vi "Wind Farm #3.vi"(8 "error in (no error)":errorcluster) -> (0 "error out":errorcluster)   [LabVIEW 2011]
doc: "This is one of 4 potential implementations for the Wind Farm Requirements. Specifically note how the wind turbine information is displayed. Also note how the main VI communicates back and forth to the wind turbine. What does that pipeline look like? Finally note the mechanism for stopping the wind turbine.\n\nAAL 9/09"
uses:
  Controls/File Type.ctl
  Controls/TYPE FGV User Event Method.ctl
  SEQ Solution/Controls/Wind Turbine DataRef.ctl
  SEQ Solution/Controls/Wind Turbine Data.ctl
  Shared/QDMH Poly VIs/QDMH POLY Enqueue String.vi
  SEQ Solution/SEQ - Solution.lvlib
panel:
  out "Wind Turbine Data":string[][](table)
  in  "File Type":T1 caption="File Type (Read When Turbine is Added)"
  in  "Set Wind Speed":bool
  in  "Wind Speed":dbl=15.0
  in  "Wind Turbine Selection":u16(ring)
  in  "Queue Name":string
  in  "Add Wind Turbine":bool
  out "Message Display":string
  in  "Exit":bool
  # "Rotation (RPM)"
  # "Wind Speed (m/s)"
  # "Running Time (sec)"
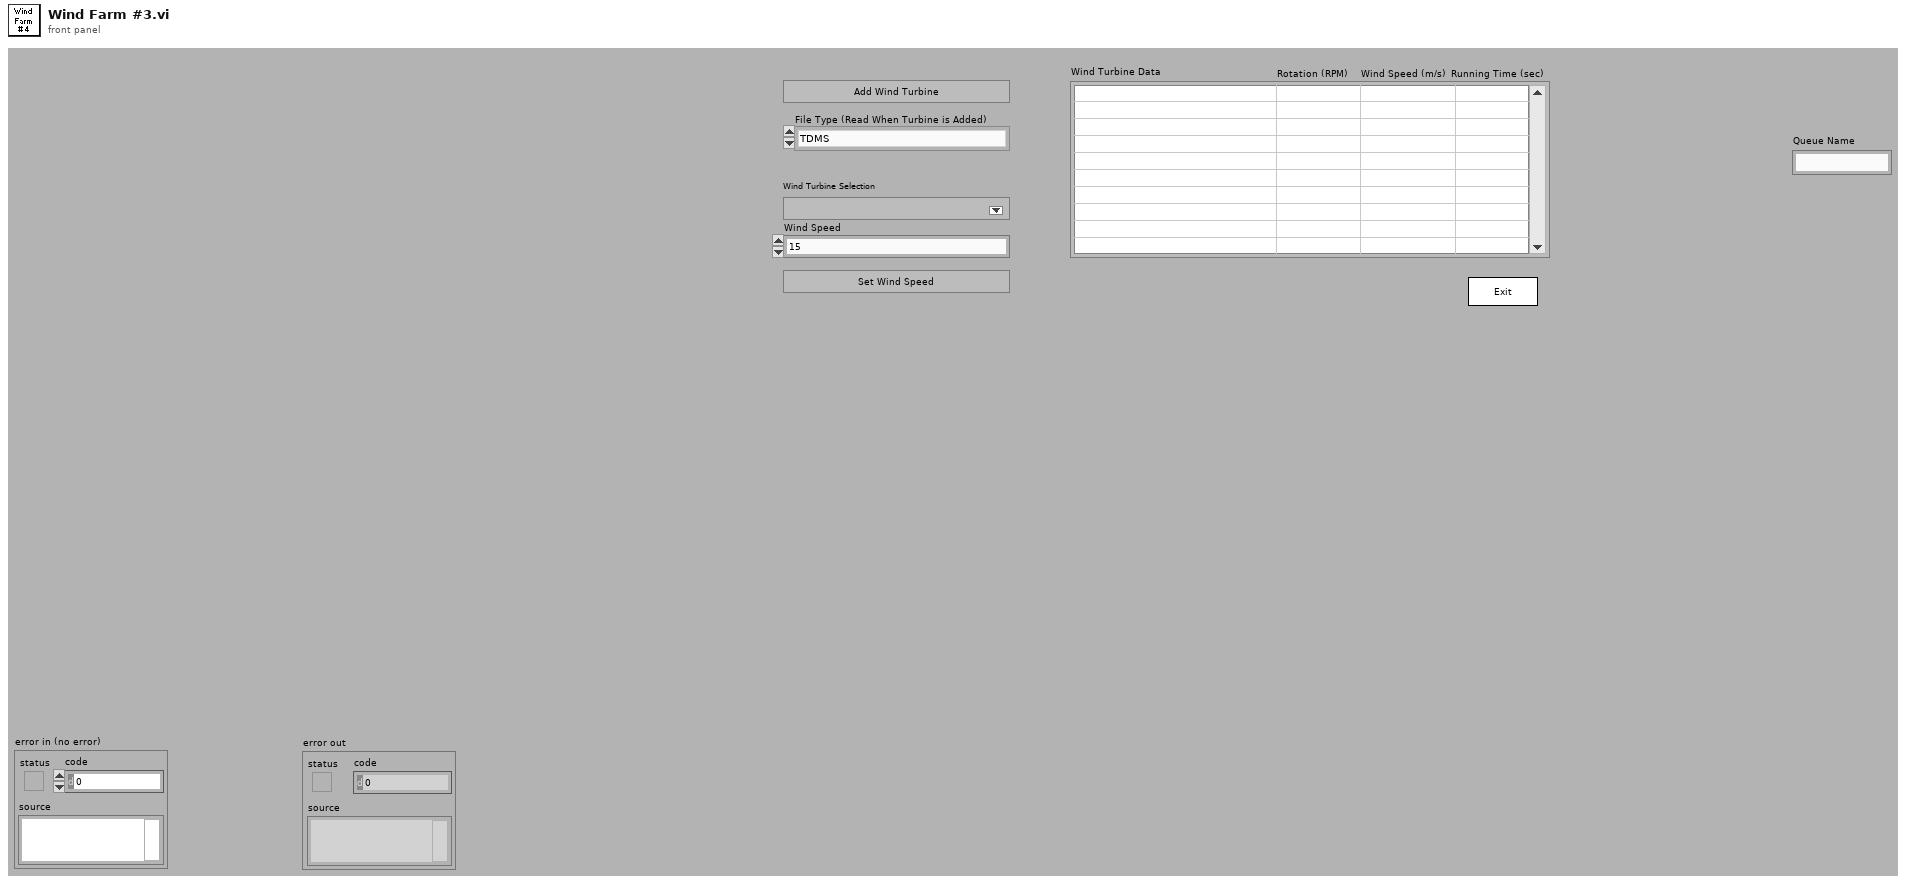
[diagram p1: front panel]
types:
  T1 = typedef "File Type.ctl" = enum16{"TDMS", "TXT"}
  T2 = typedef "TYPE FGV User Event Method.ctl" = enum16{"Add User Event Ref", "Modify User Event Ref", "Get User Event Ref", "Delete User Event Ref", "Get All User Event Refs", "Delete All User Event Refs"}
  T3 = typedef "SEQ - Solution.lvlib/Wind Turbine DataRef.ctl" = refnum<queue>
  T4 = cluster{"Operator Name":string, "Current VI's  Path":path, "Main Directory":path, "Y Data":dbl[], "Ini Path":path, "Model":string, "VITs Directory":path, "Windmill Selection":i32, "VIT References":refnum<vi>[], "VIT Current":refnum<vi>, "VIT Item Names":string[], "Wind Speed":dbl, "SEQ Wind Turbine Refs":T3[], "Timer References":refnum<data-value>[]}
  T5 = typedef "TYPE FGV User Event Ref.ctl" = refnum<user-event>
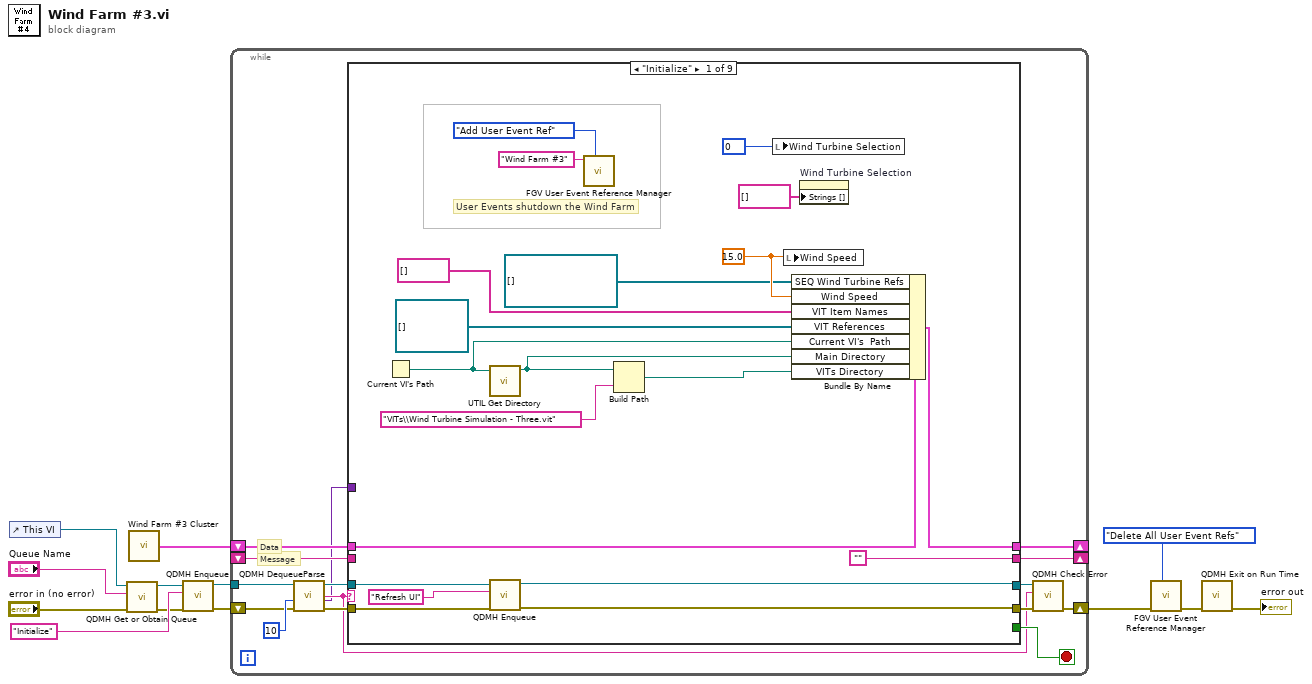
[diagram p0: block diagram]
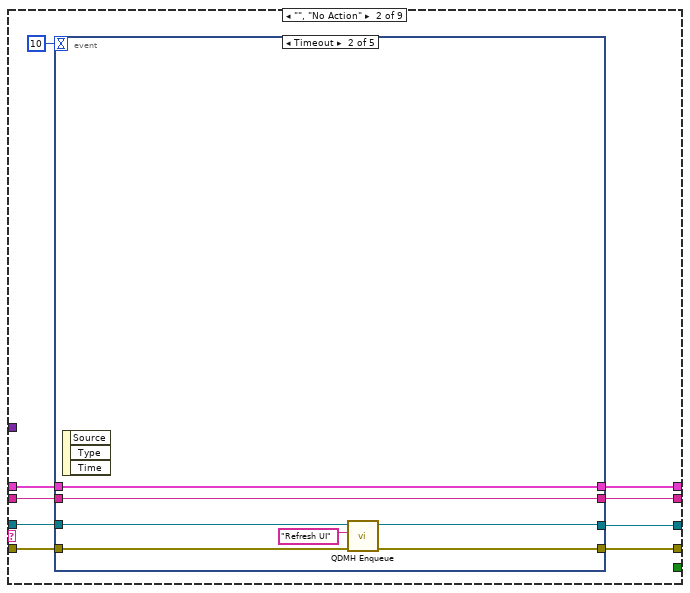
[diagram p2: hidden frame]
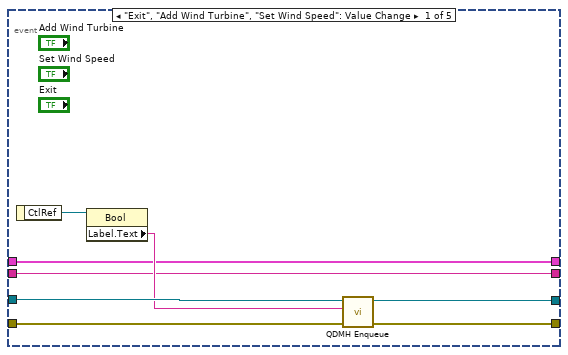
[diagram p3: hidden frame]
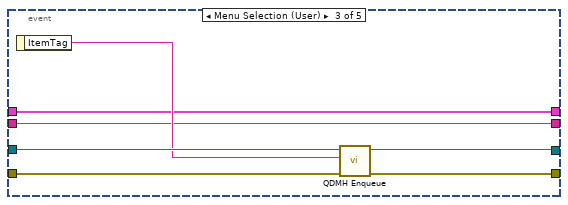
[diagram p4: hidden frame]
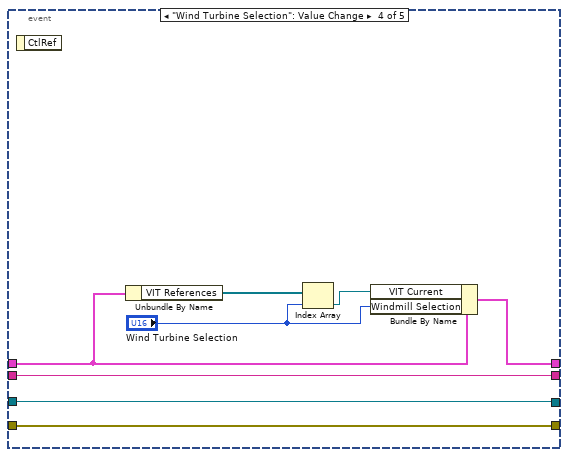
[diagram p5: hidden frame]
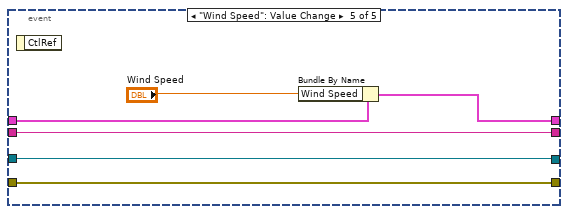
[diagram p6: hidden frame]
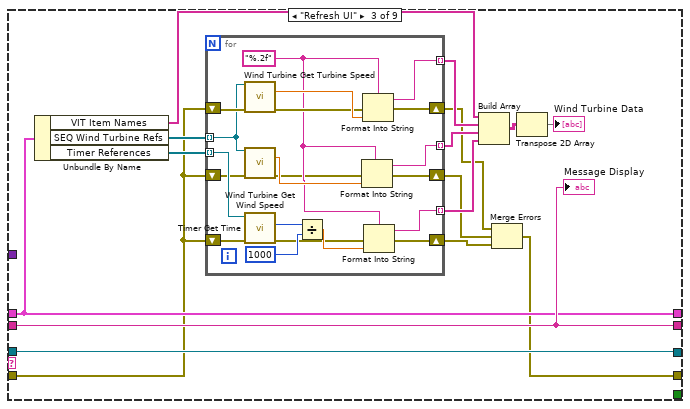
[diagram p7: hidden frame]
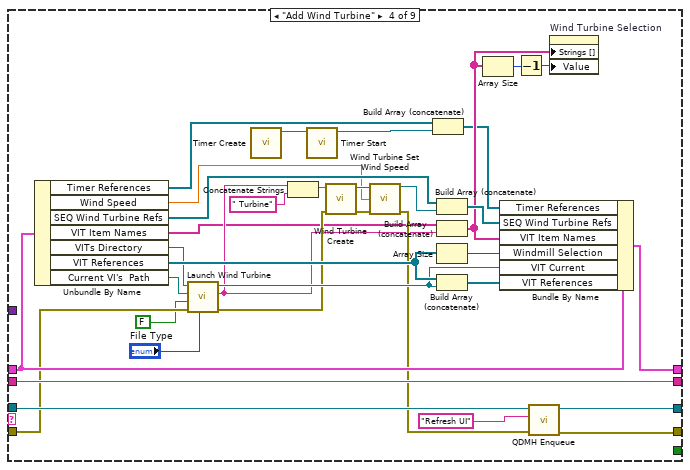
[diagram p8: hidden frame]
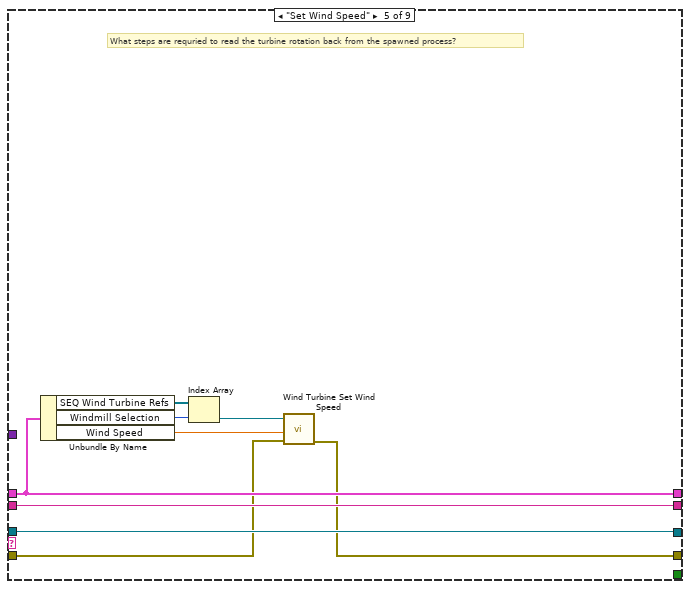
[diagram p9: hidden frame]
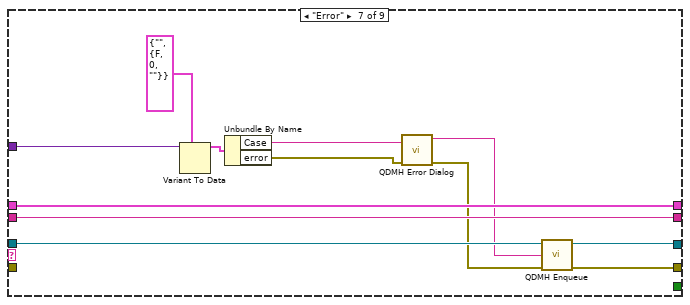
[diagram p11: hidden frame]
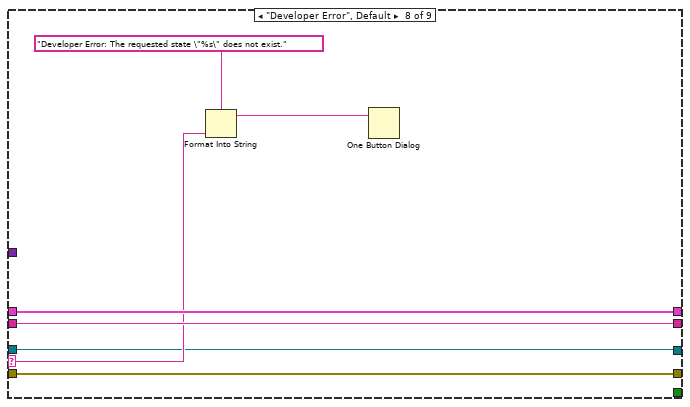
[diagram p12: hidden frame]
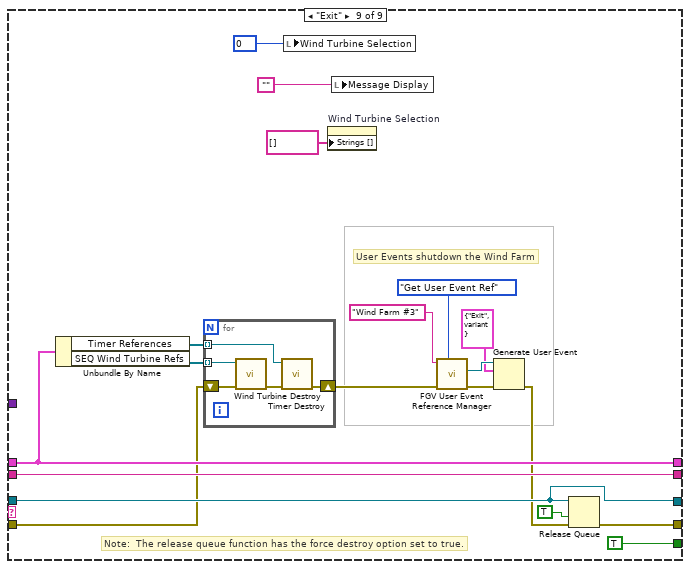
[diagram p13: hidden frame]
diagram:
  n1 = control-ref of="This VI"() -> (w4:refnum<vi>)
  n2 = call "QDMH Get or Obtain Queue.vi"("error in (no error)"="error in (no error)", "Queue Name"="Queue Name", "VI Refnum"=w4) -> ("error out"=w9:errorcluster, "queue out"=w12:refnum<queue>)  [unwired: 7 out]
  n3 = call "Wind Farm #3 Cluster.vi"() -> ("Cluster"=w6:T4)
  n4 = call-poly "QDMH Enqueue.vi"("error in (no error)"=w9, "State"="Initialize" ("element"), "queue"=w12) -> ("error out"=w10:errorcluster, "queue out"=w13:refnum<queue>)  [unwired: 7 out]
  n5 = while {
    tunnel: w13 -> [w23]
    shift-left: w6 -> [w24]
    shift-right: [w25] -> _
    shift-left: _ -> [w26]
    shift-right: [w27] -> _
    shift-right: [w17] -> w2
    shift-left: w10 -> [w19]
    stop <- w28 stop-if-true
    # "Data"
    # "Message"
    n6 = call "QDMH DequeueParse.vi"("error in (no error)"=w19, "Timeout"=10 ("ms timeout (-1)"), "queue"=w23) -> ("error out"=w20:errorcluster, "Variant Data"=w14:variant, "State"=w15:string, "queue out"=w21:refnum<queue>)  [unwired: 5 out]
    n7 = case shown="\"Initialize\"" w15 {
      selector: w15 -> [_ _ _ _ _ _ _ w193 _]
      tunnel: w21 -> [w45 w57 w108 w158 w169 w174 w187 w190 w202]
      tunnel: [_ _ _ _ _ _ _ _ TRUE] -> w28
      tunnel: ["" w50 w109 w164 w173 w177 w189 w196 w214] -> w27
      tunnel: w26 -> [_ w51 w109 w164 w173 w177 w189 w196 w214]
      tunnel: [w47 w52 w107 w161 w172 w176 w188 w195 w210] -> w25
      tunnel: w24 -> [w48 w53 w107 w162 w172 w176 w188 w195 w210]
      tunnel: w20 -> [w44 w56 w94 w151 w167 w175 _ w192 w200]
      tunnel: [w43 w55 w95 w159 w165 w175 w186 w192 w212] -> w18
      tunnel: [w36 w49 w108 w157 w169 w174 w185 w190 w202] -> w16
      tunnel: w14 -> [_ _ _ _ _ _ w180 _ _]
      frame "Initialize" {
        w35 = u16 0 items=[""] ("1 Windmill Selection")
        w34 = 15.0 ("1 Wind Speed")
        # "User Events shutdown the Wind Farm"
        n8 = Current VI's Path() -> (path=w41:path)
        n9 = call "UTIL Get Directory.vi"("Path In"=w41) -> ("Directory Out"=w40:path)  [unwired: 1 in, 9 out]
        n10 = call-poly "QDMH Enqueue.vi"("error in (no error)"=w44, "State"="Refresh UI" ("element"), "queue"=w45) -> ("error out"=w43:errorcluster, "queue out"=w36:refnum<queue>)  [unwired: 7 out]
        n11 = call "FGV User Event Reference Manager.vi"("Method (Get User Event Ref)"=TYPE_FGV_User_Event_Method."Add User Event Ref", "User Event Name"="Wind Farm #3") -> ()  [unwired: 6 in, 4 out]
        n12 = Build Path(base path=w40, name or relative path="VITs\\Wind Turbine Simulation - Three.vit") -> (appended path=w39:path)
        n13 = local write "Wind Turbine Selection"(w35) -> ()
        n14 = local write "Wind Speed"(w34) -> ()
        n15 = Bundle By Name(cluster=w48, "SEQ Wind Turbine Refs"=T3[] [], "Wind Speed"=w34, "VIT Item Names"=string[] [] ("1 VIT Item Names"), "VIT References"=refnum<vi>[] [], "Current VI's  Path"=w41, "Main Directory"=w40, "VITs Directory"=w39) -> (w47:T4)
        n16 = property on="Wind Turbine Selection" class="Ring (strict)"("Strings []"=string[] []) -> ()  [unwired: 2 in, 2 out]
      }
      frame "", "No Action" {
        n17 = event shown="[1] Timeout" {
          selector: _ -> [_ _ _ _ _]
          dyn-events: _ -> [_ _ _ _ _]
          timeout: 10 -> [_ _ _ _ _]
          tunnel: w57 -> [w64 w70 w79 w81 w90]
          tunnel: [w63 w67 w77 w80 w89] -> w55
          tunnel: w56 -> [w62 w69 w78 w80 w89]
          tunnel: w53 -> [w60 w72 w75 w84 w92]
          tunnel: [w60 w72 w75 w83 w91] -> w52
          tunnel: w51 -> [w59 w71 w74 w87 w93]
          tunnel: [w59 w71 w74 w87 w93] -> w50
          tunnel: [w58 w68 w73 w81 w90] -> w49
          event "Exit", "Add Wind Turbine", "Set Wind Speed": Value Change {
            n18 = event-data() -> ("CtlRef"=w65:refnum<vi>)  [unwired: 1 out]
            n19 = property class="Bool"(reference=w65) -> ("Label.Text"=w61:string)  [unwired: 1 in, 2 out]
            n20 = call-poly "QDMH Enqueue.vi"("error in (no error)"=w62, "State"=w61, "queue"=w64) -> ("error out"=w63:errorcluster, "queue out"=w58:refnum<queue>)  [unwired: 7 out]
          }
          event Timeout {
            n21 = event-data() -> ()  [unwired: 4 out]
            n22 = call-poly "QDMH Enqueue.vi"("error in (no error)"=w69, "State"="Refresh UI", "queue"=w70) -> ("error out"=w67:errorcluster, "queue out"=w68:refnum<queue>)  [unwired: 7 out]
          }
          event Menu Selection (User) {
            n23 = event-data() -> ("ItemTag"=w76:string)  [unwired: 1 out]
            n24 = call-poly "QDMH Enqueue.vi"("error in (no error)"=w78, "State"=w76, "queue"=w79) -> ("error out"=w77:errorcluster, "queue out"=w73:refnum<queue>)  [unwired: 7 out]
          }
          event "Wind Turbine Selection": Value Change {
            n25 = event-data() -> ()  [unwired: 2 out]
            n26 = Unbundle By Name(w84) -> ("VIT References"=w86:refnum<vi>[])
            n27 = Index Array(array=w86, index="Wind Turbine Selection") -> (element=w85:refnum<vi>)
            n28 = Bundle By Name(cluster=w84, "VIT Current"=w85, "Windmill Selection"="Wind Turbine Selection") -> (w83:T4)
          }
          event "Wind Speed": Value Change {
            n29 = event-data() -> ()  [unwired: 2 out]
            n30 = Bundle By Name(cluster=w92, "Wind Speed"="Wind Speed") -> (w91:T4)
          }
        }
      }
      frame "Refresh UI" {
        n31 = Unbundle By Name(w107) -> ("VIT Item Names"=w102:string[], "SEQ Wind Turbine Refs"=w101:T3[], "Timer References"=w106:refnum<data-value>[])
        n32 = for {
          tunnel: w106 -> [w123] mode=indexing
          tunnel: [w128] -> w105 mode=indexing
          shift-right: [w120] -> w98
          shift-left: w94 -> [w122]
          tunnel: w101 -> [w116] mode=indexing
          tunnel: [w124] -> w99 mode=indexing
          shift-right: [w117] -> w96
          shift-left: w94 -> [w119]
          shift-right: [w111] -> w97
          shift-left: w94 -> [w113]
          tunnel: [w110] -> w100 mode=indexing
          w114 = "%.2f" ("format string")
          n33 = call "Wind Turbine Get Turbine Speed.vi"("Data Refnum"=w116, "error in (no error)"=w122) -> ("Turbine Speed (RPM)"=w129:dbl, "error out"=w121:errorcluster)  [unwired: 11 in, 1 out]
          n34 = call "Wind Turbine Get Wind Speed.vi"("Data Refnum"=w116, "error in (no error)"=w113) -> ("Wind Speed (M/s)"=w115:dbl, "error out"=w112:errorcluster)  [unwired: 11 in, 1 out]
          n35 = call "Timer Get Time.vi"("error in (no error)"=w119, "Timer reference"=w123) -> ("error out"=w118:errorcluster, "Elapsed Time (ms)"=w127:u32)  [unwired: 6 in, 2 out]
          n36 = Divide(x=w127, y=u32 1000) -> (x/y=w125:dbl)
          n37 = Format Into String(format string=w114, error in=w112, w115) -> (resulting string=w110:string, error out=w111:errorcluster)  [unwired: 1 in]
          n38 = Format Into String(format string=w114, error in=w121, w129) -> (resulting string=w128:string, error out=w120:errorcluster)  [unwired: 1 in]
          n39 = Format Into String(format string=w114, error in=w118, w125) -> (resulting string=w124:string, error out=w117:errorcluster)  [unwired: 1 in]
        }
        n40 = Build Array(w102, w105, w100, w99) -> (w104:string[][])
        n41 = Merge Errors(w98, w97, w96) -> (w95:errorcluster)
        n42 = Transpose 2D Array(2D array=w104) -> (transposed array=→"Wind Turbine Data":string[][])
        "Message Display" <- w109
      }
      frame "Add Wind Turbine" {
        n43 = Unbundle By Name(w162) -> ("Timer References"=w130:refnum<data-value>[], "Wind Speed"=w141:dbl, "SEQ Wind Turbine Refs"=w150:T3[], "VIT Item Names"=w137:string[], "VITs Directory"=w155:path, "VIT References"=w156:refnum<vi>[], "Current VI's  Path"=w154:path)
        n44 = call "Launch Wind Turbine.vi"("File Type"="File Type", "error in"=w151, "Front Panel Open?"=FALSE, "Calling VI Path"=w154, "VIT Path"=w155) -> ("error out"=w144:errorcluster, "Name"=w139:string, "vi reference"=w153:refnum<vi>)  [unwired: 4 in]
        n45 = call "Timer Create.vi"() -> ("Timer reference out"=w133:refnum<data-value>)  [unwired: 10 in, 1 out]
        n46 = Concatenate Strings(w139, " Turbine" ("string")) -> (w138:string)
        n47 = call "Timer Start.vi"("Timer reference"=w133) -> ("Timer reference  out"=w132:refnum<data-value>)  [unwired: 9 in, 1 out]
        n48 = call "Wind Turbine Create.vi"("error in (no error)"=w144, "SEQ Name"=w138) -> ("error out"=w142:errorcluster, "Data Refnum out"=w146:T3)  [unwired: 8 in]
        n49 = call "Wind Turbine Set Wind Speed.vi"("Data Refnum"=w146, "Wind Speed (ms)"=w141, "error in (no error)"=w142) -> ("Data Refnum out"=w145:T3, "error out"=w143:errorcluster)  [unwired: 11 in]
        n50 = Build Array (concatenate)(w130, w132) -> (w131:refnum<data-value>[])
        n51 = Build Array (concatenate)(w150, w145) -> (w149:T3[])
        n52 = Build Array (concatenate)(w137, w139) -> (w134:string[])
        n53 = Array Size(array=w156) -> (size(s)=w147:i32)
        n54 = Build Array (concatenate)(w156, w153) -> (w163:refnum<vi>[])
        n55 = Array Size(array=w134) -> (size(s)=w136:i32)
        n56 = Bundle By Name(cluster=w162, "Timer References"=w131, "SEQ Wind Turbine Refs"=w149, "VIT Item Names"=w134, "Windmill Selection"=w147, "VIT Current"=w153, "VIT References"=w163) -> (w161:T4)
        n57 = Decrement(x=w136) -> (x-1=w135:i32)
        n58 = call-poly "QDMH Enqueue.vi"("error in (no error)"=w143, "State"="Refresh UI" ("element"), "queue"=w158) -> ("error out"=w159:errorcluster, "queue out"=w157:refnum<queue>)  [unwired: 7 out]
        n59 = property on="Wind Turbine Selection" class="Ring (strict)"("Strings []"=w134, "Value"=w135) -> ()  [unwired: 2 in, 2 out]
      }
      frame "Set Wind Speed" {
        # "What steps are requried to read the turbine rotation back from the spawned process?"
        n60 = Unbundle By Name(w172) -> ("SEQ Wind Turbine Refs"=w171:T3[], "Windmill Selection"=w170:i32, "Wind Speed"=w166:dbl)
        n61 = Index Array(array=w171, index=w170) -> (element=w168:T3)
        n62 = call "Wind Turbine Set Wind Speed.vi"("Data Refnum"=w168, "Wind Speed (ms)"=w166, "error in (no error)"=w167) -> ("error out"=w165:errorcluster)  [unwired: 11 in, 1 out]
      }
      frame "<add states as needed>" {
        # "Duplicate this state for any additional states that you add."
      }
      frame "Error" {
        n63 = Variant To Data(type=cluster{"Case":string, "error":errorcluster} {"Case"="", "error"={"status"=FALSE, "code"=0, "source"=""}} ("QDSM Element"), Variant=w180) -> (data=w183:cluster{"Case":string, "error":errorcluster})  [unwired: 1 in, 1 out]
        n64 = Unbundle By Name(w183) -> ("Case"=w182:string, "error"=w181:errorcluster)
        n65 = call "QDMH Error Dialog.vi"("error"=w181, "Case Error Occured"=w182) -> ("error out (no error)"=w178:errorcluster, "Case to Execute"=w179:string)  [unwired: 8 out]
        n66 = call-poly "QDMH Enqueue.vi"("error in (no error)"=w178, "State"=w179, "queue"=w187) -> ("error out"=w186:errorcluster, "queue out"=w185:refnum<queue>)  [unwired: 7 out]
      }
      frame "Developer Error", Default {
        n67 = Format Into String(format string="Developer Error: The requested state \"%s\" does not exist." ("message"), w193) -> (resulting string=w191:string)  [unwired: 2 in, 1 out]
        n68 = One Button Dialog(message=w191) -> ()  [unwired: 2 out]
      }
      frame "Exit" {
        w208 = u16 0 items=[""] ("1 Windmill Selection")
        # "User Events shutdown the Wind Farm"
        # "Note:  The release queue function has the force destroy option set to true."
        n69 = Unbundle By Name(w210) -> ("Timer References"=w197:refnum<data-value>[], "SEQ Wind Turbine Refs"=w207:T3[])
        n70 = for {
          tunnel: w207 -> [w220] mode=indexing
          shift-right: [w216] -> w201
          shift-left: w200 -> [w219]
          tunnel: w197 -> [w218] mode=indexing
          n71 = call "Wind Turbine Destroy.vi"("error in (no error)"=w219, "Data Refnum"=w220) -> ("error out"=w217:errorcluster)  [unwired: 8 in, 1 out]
          n72 = call "Timer Destroy.vi"("error in (no error)"=w217, "Timer reference"=w218) -> ("error out"=w216:errorcluster)  [unwired: 9 in]
        }
        n73 = local write "Wind Turbine Selection"(w208) -> ()
        n74 = property on="Wind Turbine Selection" class="Ring (strict)"("Strings []"=string[] []) -> ()  [unwired: 2 in, 2 out]
        n75 = local write "Message Display"("") -> ()
        n76 = call "FGV User Event Reference Manager.vi"("Method (Get User Event Ref)"=TYPE_FGV_User_Event_Method."Get User Event Ref", "error in (no error)"=w201, "User Event Name"="Wind Farm #3") -> ("error out"=w204:errorcluster, "User Event Ref  Out"=w203:T5)  [unwired: 5 in, 2 out]
        n77 = Generate User Event(user event=w203, event data cluster=cluster{"String":string, "Data":variant} {"String"="Exit", "Data"=variant} ("event data"), error in=w204) -> (error out=w199:errorcluster)  [unwired: 1 out]
        n78 = Release Queue(queue=w202, force destroy? (F)=TRUE, error in (no error)=w199) -> (error out=w212:errorcluster)  [unwired: 2 out]
      }
    }
    n79 = call "QDMH Check Error.vi"("error in (no error)"=w18, "Case"=w15, "queue"=w16) -> ("error out"=w17:errorcluster)  [unwired: 1 in, 7 out]
  }
  n80 = call "FGV User Event Reference Manager.vi"("Method (Get User Event Ref)"=TYPE_FGV_User_Event_Method."Delete All User Event Refs", "error in (no error)"=w2) -> ("error out"=w1:errorcluster)  [unwired: 6 in, 3 out]
  n81 = call "QDMH Exit on Run Time.vi"("error in (no error)"=w1) -> ("error out"=→"error out":errorcluster)  [unwired: 10 out]
